vi "Set A Bit U64.vi"(9 "Input":u64 format="%08x", 10 "B":bool, 11 "Bit Number":u64) -> (3 "Output":u64 format="%08x")   [LabVIEW 2021]
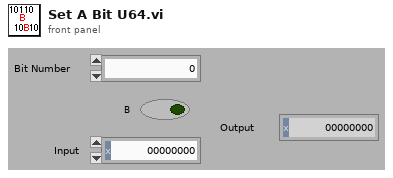
[diagram p1: front panel]
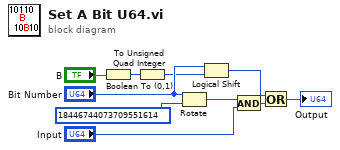
[diagram p0: block diagram]
diagram:
  n1 = Boolean To (0,1)(Boolean="B") -> (0, 1=w6:i16)
  n2 = To Unsigned Quad Integer(1:w6) -> (0:w2:u64)
  n3 = Rotate(1:u64 18446744073709551614 ("x"), 2:"Bit Number") -> (0:w1:u64)
  n4 = Logical Shift(y="Bit Number", x=w2) -> (x << y=w3:u64)
  n5 = And(x=w1, y="Input") -> (x .and. y?=w8:u64)
  n6 = Or(x=w3, y=w8) -> (x .or. y?=→"Output":u64)
